vi "Checkers Load Game.vi"   [LabVIEW 2016]
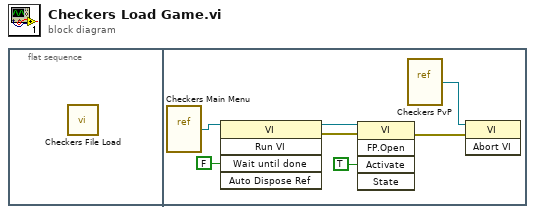
[diagram p0: block diagram]
diagram:
  n1 = flat-sequence {
    frame #0 {
      n2 = call "Checkers File Load.vi"() -> ()  [unwired: 12 in]
    }
    frame #1 {
      n3 = vi-ref "Checkers Main Menu.vi"() -> (w1:refnum<vi>)
      n4 = invoke class="VI" method="Run VI"(reference=w1, "Wait until done"=FALSE ("Wait Until Done")) -> (reference out=w2:refnum<vi>, error out=w3:errorcluster)  [unwired: 3 in, 3 out]
      n5 = invoke class="VI" method="FP.Open"(reference=w2, error in=w3, "Activate"=TRUE ("Activate?")) -> (error out=w4:errorcluster)  [unwired: 2 in, 4 out]
      n6 = vi-ref "Checkers PvP.vi"() -> (w5:refnum<vi>)
      n7 = invoke class="VI" method="Abort VI"(reference=w5, error in=w4) -> ()  [unwired: 1 in, 3 out]
    }
  }
